vi "Read Charge Pump Information.vi"(11 "Toggle 6 in":refnum<class "Toggle 6.lvclass">) -> (2 "Charge Pump Information":T1={"Min"=29.75, "Max"=50.0, "Step"=0.75, "Default"=0.75}, 3 "Toggle 6 out":refnum<class "Toggle 6.lvclass">)   [LabVIEW 2020, in "Toggle 6.lvclass"]
uses:
  Toggle 6.lvclass
  Controls/Charge Pump Information cluster.ctl
  Toggle 6.lvclass/Toggle 6.ctl
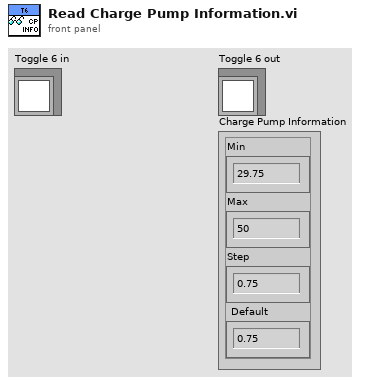
[diagram p1: front panel]
types:
  T1 = typedef "Toggle 6.lvclass/Charge Pump Information cluster.ctl" = cluster{"Min":dbl, "Max":dbl, "Step":dbl, "Default":dbl}
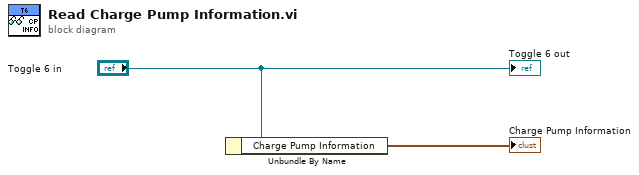
[diagram p0: block diagram]
diagram:
  n1 = Unbundle By Name("Toggle 6 in") -> ("Charge Pump Information"=→"Charge Pump Information":T1)
  "Toggle 6 out" <- "Toggle 6 in"
